vi "1D数组排序[CSG 幅度,实部,虚部].vi"(8 "error in (no error)":errorcluster caption="错误输入（无错误）", 9 "升降序":enum16{"升序", "降序"}(ring), 11 "输入数组":csg[](array[numeric])) -> (0 "error out":errorcluster caption="错误输出", 2 "排序后索引":i32[](array[numeric]), 3 "排序后数组":csg[](array[numeric]) format="%.2f")   [LabVIEW 2018]
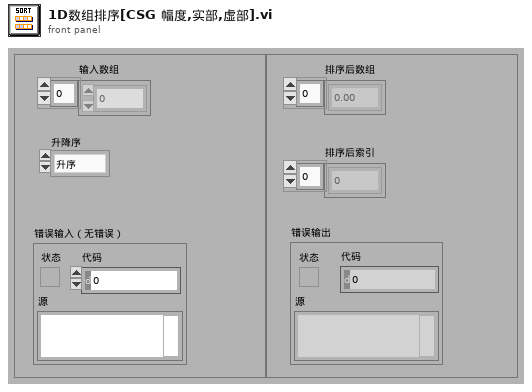
[diagram p1: front panel]
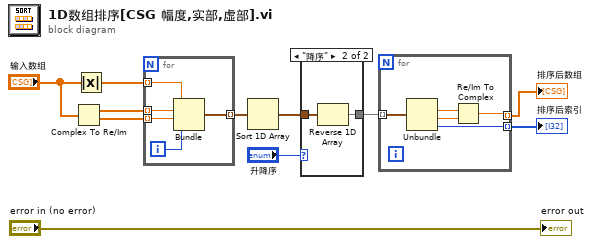
[diagram p0: block diagram]
diagram:
  n1 = Complex To Re/Im(x + iy="输入数组") -> (x=w8:sgl[], y=w7:sgl[])
  n2 = Absolute Value(x="输入数组") -> (abs(x)=w10:sgl[])
  n3 = for {
    tunnel: [w16] -> w9 mode=indexing
    tunnel: w10 -> [w15] mode=indexing
    tunnel: w8 -> [w14] mode=indexing
    tunnel: w7 -> [w13] mode=indexing
    i -> [w12]
    n4 = Bundle("数值"=w15, "数值"=w14, "数值"=w13, w12) -> (w16:cluster{"数值":sgl, "数值":sgl, "数值":sgl, i32})  [unwired: 1 in]
  }
  n5 = Sort 1D Array(array=w9) -> (sorted array=w2:cluster{"数值":sgl, "数值":sgl, "数值":sgl, i32}[])
  n6 = case shown="\"降序\"" "升降序" {
    tunnel: w2 -> [w17 w19]
    tunnel: [w17 w18] -> w1
    frame "升序", Default {
    }
    frame "降序" {
      n7 = Reverse 1D Array(array=w19) -> (reversed array=w18:cluster{"数值":sgl, "数值":sgl, "数值":sgl, i32}[])
    }
  }
  n8 = for {
    tunnel: w1 -> [w24] mode=indexing
    tunnel: [w21] -> w6 mode=indexing
    tunnel: [w20] -> w5 mode=indexing
    n9 = Unbundle(w24) -> ("数值"=w22:sgl, "数值"=w23:sgl, w20:i32)  [unwired: 1 out]
    n10 = Re/Im To Complex(1:w23, 2:w22) -> (0:w21:csg)
  }
  "排序后数组" <- w6
  "排序后索引" <- w5
  "error out" <- "error in (no error)"
